vi "히로시마_TEST.vi"() -> ()   [LabVIEW 2023]
uses:
  <vilib>/Analysis/2dsp.llb/Complex FFT.vi
  <vilib>/Analysis/2dsp.llb/Real FFT.vi
  <vilib>/Analysis/NI_AALBase.lvlib
  <vilib>/Analysis/NI_AALPro.lvlib
panel:
  in  "amplitude":dbl=1.0 caption="진폭" format="%0.2f"
  out "웨이브폼 그래프 4":waveform(dbl)(graph)
  out "웨이브폼 그래프 3":waveform(dbl)(graph)
  out "웨이브폼 그래프 5":waveform(dbl)(graph)
  in  "수신시간":dbl=5500.0 format="%#_13g"
  in  "위상":dbl=5500.0 format="%#_13g"
  in  "Fs":dbl=5500.0 format="%#_13g"
  in  "주파수":dbl=5500.0 format="%#_13g"
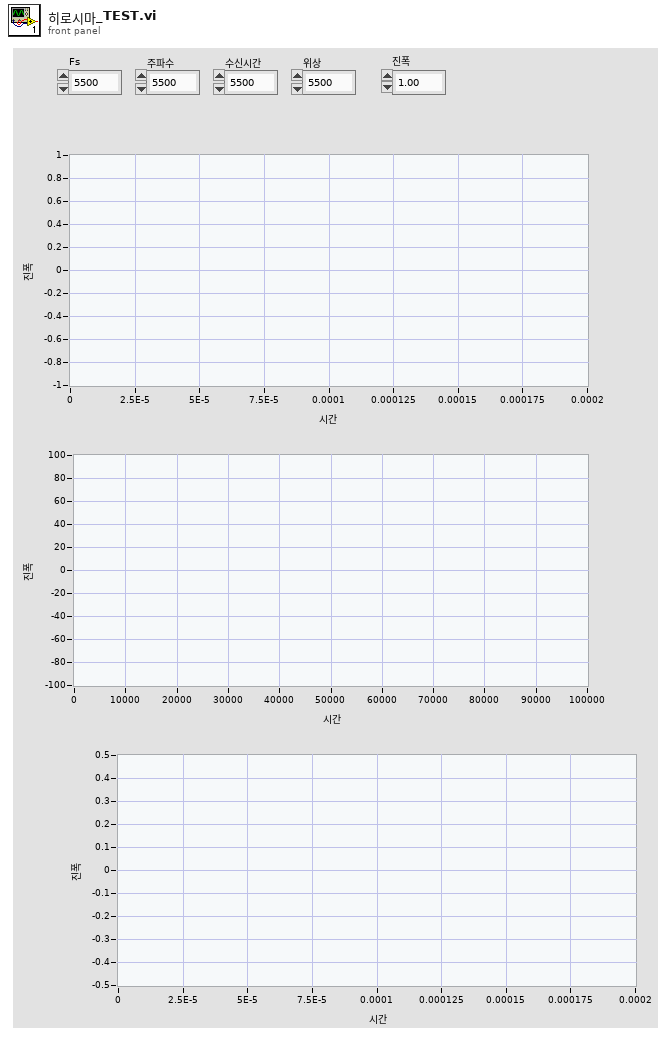
[diagram p1: front panel]
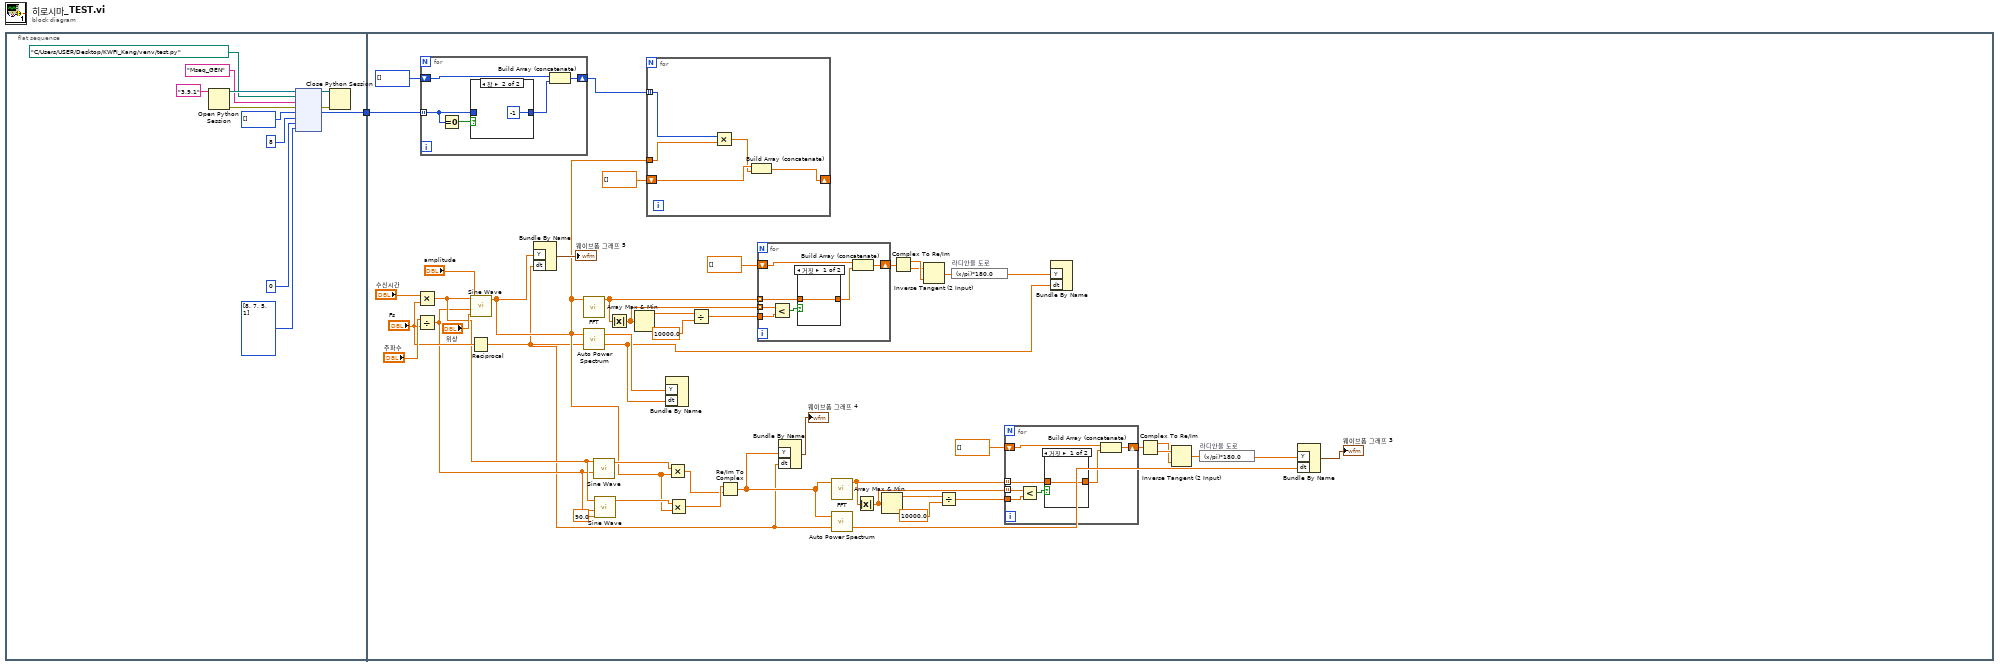
[diagram p0: block diagram]
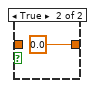
[diagram p2: hidden frame]
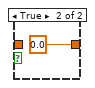
[diagram p3: hidden frame]
diagram:
  n1 = flat-sequence {
    tunnel: [w2] -> w1
    tunnel: w1 -> [w58]
    frame #0 {
      n2 = Open Python Session(python version="3.9.1" ("Python 버전")) -> (session out=w12:refnum<k35>, error out=w11:errorcluster)  [unwired: 2 in]
      n3 = node(w12, path "C:/Users/USER/Desktop/KWFI_Kang/venv/test.py" ("Python 경로"), "Mseq_GEN" ("함수 이름"), w11, i32[] [], 8, 0, i32[] [8, 7, 5, 1]) -> (w9:refnum<k35>, w10:errorcluster, w2:i32[])  [unwired: 3 in, 2 out]
      n4 = Close Python Session(session in=w9, error in=w10) -> ()  [unwired: 1 out]
    }
    frame #1 {
      n5 = Multiply(x="수신시간", y="Fs") -> (x*y=w40:dbl)
      n6 = Divide(x="주파수", y="Fs") -> (x/y=w39:dbl)
      n7 = for {
        tunnel: w58 -> [w85] mode=indexing
        shift-right: [w84] -> w42
        shift-left: i32[] [] -> [w87]
        n8 = Equal To 0?(x=w85) -> (x = 0?=w88:bool)
        n9 = case shown="참" w88 {
          tunnel: [w89 -1] -> w86
          tunnel: w85 -> [w89 _]
          frame False {
          }
          frame True {
          }
        }
        n10 = Build Array (concatenate)(w87, w86) -> (w84:i32[])
      }
      n11 = Reciprocal(x="Fs") -> (1/x=w16:dbl)
      n12 = call <vilib>:"Sine Wave.vi"("samples"=w40, "amplitude"="amplitude", "frequency"=w39, "phase in"="위상") -> ("sine wave"=w34:dbl[])  [unwired: 1 in, 2 out]
      n13 = Bundle By Name("Y"=w34, "dt"=w16) -> (→"웨이브폼 그래프 5":waveform(dbl))  [unwired: 1 in]
      n14 = call-poly <vilib>:"FFT.vi"("X"=w34) -> ("FFT {X}"=w53:cdb[])  [unwired: 9 in, 1 out]
      n15 = call <vilib>:"Auto Power Spectrum.vi"("dt"=w16, "Signal (V)"=w34) -> ("df"=w33:dbl, "Power Spectrum (V^2 rms)"=w43:dbl[])
      n16 = call <vilib>:"Sine Wave.vi"("samples"=w40, "frequency"=w39) -> ("sine wave"=w37:dbl[])  [unwired: 3 in, 2 out]
      n17 = call <vilib>:"Sine Wave.vi"("samples"=w40, "frequency"=w39, "phase in"=90.0) -> ("sine wave"=w36:dbl[])  [unwired: 2 in, 2 out]
      n18 = Absolute Value(x=w53) -> (abs(x)=w52:dbl[])
      n19 = Array Max & Min(array=w52) -> (max value=w55:dbl)  [unwired: 3 out]
      n20 = for {
        tunnel: w34 -> [w73]
        tunnel: w42 -> [w74] mode=indexing
        shift-right: [w70] -> _
        shift-left: dbl[] [] -> [w72]
        n21 = Multiply(x=w74, y=w73) -> (x*y=w71:dbl[])
        n22 = Build Array (concatenate)(w72, w71) -> (w70:dbl[])
      }
      n23 = Bundle By Name("Y"=w43, "dt"=w33) -> ()  [unwired: 1 in, 1 out]
      n24 = Multiply(x=w37, y=w34) -> (x*y=w19:dbl[])
      n25 = Multiply(x=w36, y=w34) -> (x*y=w20:dbl[])
      n26 = Divide(x=w55, y=10000.0) -> (x/y=w51:dbl)
      n27 = Re/Im To Complex(1:w19, 2:w20) -> (0:w17:cdb[])
      n28 = for {
        tunnel: w53 -> [w76] mode=indexing
        tunnel: w52 -> [w81] mode=indexing
        tunnel: w51 -> [w80]
        shift-right: [w75] -> w49
        shift-left: dbl[] [] -> [w78]
        n29 = Less?(x=w81, y=w80) -> (x < y?=w79:bool)
        n30 = case shown="거짓" w79 {
          tunnel: [w82 0.0] -> w77
          tunnel: w76 -> [w82 _]
          frame False {
          }
          frame True {
          }
        }
        n31 = Build Array (concatenate)(w78, w77) -> (w75:cdb[])
      }
      n32 = Bundle By Name("Y"=w17, "dt"=w16) -> (→"웨이브폼 그래프 4":waveform(cdb))  [unwired: 1 in]
      n33 = call-poly <vilib>:"FFT.vi"("X"=w17) -> ("FFT {X}"=w23:cdb[])  [unwired: 9 in, 1 out]
      n34 = call <vilib>:"Auto Power Spectrum.vi"("dt"=w16, "Signal (V)"=w17) -> ("df"=w32:dbl)  [unwired: 1 out]
      n35 = Absolute Value(x=w23) -> (abs(x)=w24:dbl[])
      n36 = Array Max & Min(array=w24) -> (max value=w21:dbl)  [unwired: 3 out]
      n37 = Complex To Re/Im(x + iy=w49) -> (x=w48:dbl[], y=w47:dbl[])
      n38 = Inverse Tangent (2 Input)(1:w48, 2:w47) -> (0:w46:dbl[])
      n39 = Divide(x=w21, y=10000.0) -> (x/y=w25:dbl)
      n40 = expression code="(x/pi)*180.0" "라디안을 도로"(w46) -> (w44:dbl[])
      n41 = for {
        tunnel: w23 -> [w62] mode=indexing
        tunnel: w24 -> [w67] mode=indexing
        tunnel: w25 -> [w66]
        shift-right: [w61] -> w27
        shift-left: dbl[] [] -> [w64]
        n42 = Less?(x=w67, y=w66) -> (x < y?=w65:bool)
        n43 = case shown="거짓" w65 {
          tunnel: [w68 0.0] -> w63
          tunnel: w62 -> [w68 _]
          frame False {
          }
          frame True {
          }
        }
        n44 = Build Array (concatenate)(w64, w63) -> (w61:cdb[])
      }
      n45 = Bundle By Name("Y"=w44, "dt"=w33) -> ()  [unwired: 1 in, 1 out]
      n46 = Complex To Re/Im(x + iy=w27) -> (x=w28:dbl[], y=w29:dbl[])
      n47 = Inverse Tangent (2 Input)(1:w28, 2:w29) -> (0:w30:dbl[])
      n48 = expression code="(x/pi)*180.0" "라디안을 도로"(w30) -> (w31:dbl[])
      n49 = Bundle By Name("Y"=w31, "dt"=w32) -> (→"웨이브폼 그래프 3":waveform(dbl))  [unwired: 1 in]
    }
  }
